vi "ramp dbl.vi"(2 "ramp mode":T1(ring), 3 "initialize":cluster{"value":dbl, "reset":bool}, 4 "max change/s":dbl, 5 "setpoint":dbl(slide) scale=-1.0..1.0) -> (0 "seconds elapsed":dbl format="%.2f", 1 "output":dbl(slide) scale=-1.0..1.0)   [LabVIEW 2009]
doc: "Ramps a value or array of values. In order for the array portion to function properly, it must be initialized (so that it knows how large the array is)"
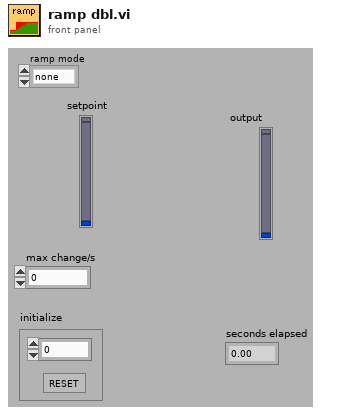
[diagram p1: front panel]
types:
  T1 = enum8{"none", "descel only", "accel only", "both"}
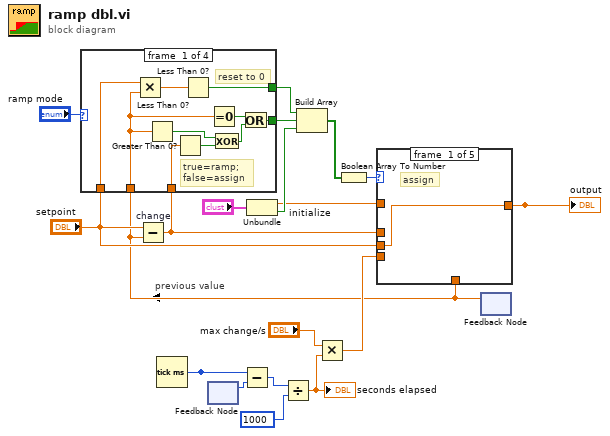
[diagram p0: block diagram]
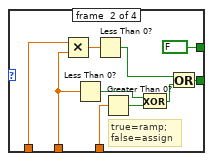
[diagram p2: hidden frame]
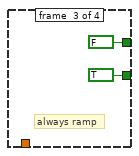
[diagram p3: hidden frame]
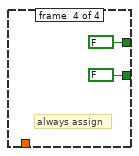
[diagram p4: hidden frame]
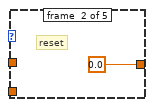
[diagram p5: hidden frame]
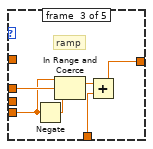
[diagram p6: hidden frame]
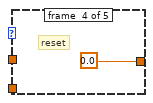
[diagram p7: hidden frame]
diagram:
  # "previous value"
  n1 = Tick Count (ms)() -> (millisecond timer value=w18:u32)
  n2 = feedback #1() -> (w19:u32)  [unwired: 1 in]
  n3 = Subtract(x=w18, y=w19) -> (x-y=w2:u32)
  n4 = Unbundle("initialize") -> ("value"=w13:dbl, "reset"=w16:bool)
  n5 = Divide(x=w2, y=u32 1000) -> (x/y=w3:dbl)
  "seconds elapsed" <- w3
  n6 = Multiply(x="max change/s", y=w3) -> (x*y=w11:dbl)
  n7 = feedback #2() -> (w7:dbl)  [unwired: 1 in]
  n8 = Subtract "change"(x="setpoint", y=w7) -> (x-y=w12:dbl)
  n9 = case shown="\"none\"" "ramp mode" {
    tunnel: w12 -> [w29 w39 _ _]
    tunnel: "setpoint" -> [w28 w38 _ _]
    tunnel: [w27 FALSE FALSE FALSE] -> w8
    tunnel: w7 -> [w26 w37 _ _]
    tunnel: [w25 w36 TRUE FALSE] -> w6
    frame #0 {
      # "reset to 0"
      # "true=ramp;\nfalse=assign"
      n10 = Multiply(x=w28, y=w26) -> (x*y=w22:dbl)
      n11 = Less Than 0?(x=w26) -> (x < 0?=w23:bool)
      n12 = Greater Than 0?(x=w29) -> (x > 0?=w24:bool)
      n13 = Less Than 0?(x=w22) -> (x < 0?=w27:bool)
      n14 = Equal To 0?(x=w26) -> (x = 0?=w21:bool)
      n15 = Exclusive Or(1:w24, 2:w23) -> (0:w20:bool)
      n16 = Or(x=w21, y=w20) -> (x .or. y?=w25:bool)
    }
    frame #1 {
      # "true=ramp;\nfalse=assign"
      n17 = Multiply(x=w38, y=w37) -> (x*y=w33:dbl)
      n18 = Less Than 0?(x=w37) -> (x < 0?=w34:bool)
      n19 = Less Than 0?(x=w33) -> (x < 0?=w30:bool)
      n20 = Greater Than 0?(x=w39) -> (x > 0?=w35:bool)
      n21 = Exclusive Or(1:w35, 2:w34) -> (0:w32:bool)
      n22 = Or(x=w30, y=w32) -> (x .or. y?=w36:bool)
    }
    frame #2 {
      # "always ramp"
    }
    frame #3 {
      # "always assign"
    }
  }
  n23 = Build Array(w8, w6, w16) -> (w15:bool[])
  n24 = Boolean Array To Number(Boolean array=w15) -> (number=w14:u32)
  n25 = case shown="2" w14 {
    tunnel: [w44 0.0 ("value") w48 0.0 w53] -> w10
    tunnel: w13 -> [_ _ _ _ w53]
    tunnel: w7 -> [_ _ w49 _ _]
    tunnel: w12 -> [_ _ w47 _ _]
    tunnel: w11 -> [_ _ w46 _ _]
    tunnel: "setpoint" -> [w44 _ _ _ _]
    frame #0 {
      # "assign"
    }
    frame #1 {
      # "reset"
    }
    frame #2 {
      # "ramp"
      n26 = Negate(x=w46) -> (-x=w51:dbl)
      n27 = In Range and Coerce(upper limit=w46, x=w47, lower limit=w51) -> (coerced(x)=w50:dbl)  [unwired: 1 out]
      n28 = Add(x=w50, y=w49) -> (x+y=w48:dbl)
    }
    frame #3 {
      # "reset"
    }
    frame #4 {
      # "initialize"
    }
  }
  "output" <- w10
